vi "Load Selected File Format Class.vi"(8 "error in (no error)":errorcluster, 10 "Protocol in":string, 11 "Class Lookup":variant) -> (0 "error out":errorcluster, 2 "FileFormat.lvclass":refnum<class "FileFormat.lvclass">, 3 "Class Lookup":variant)   [LabVIEW 2013, in "Engine Simulation Toolkit System Explorer.lvlib"]
uses:
  Engine Simulation Toolkit System Explorer.lvlib
  File Formats.lvlibp/Parent/FileFormat.lvclass
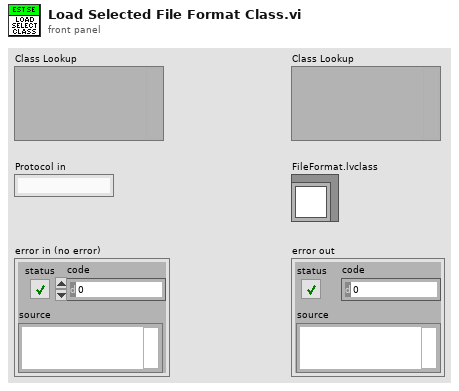
[diagram p1: front panel]
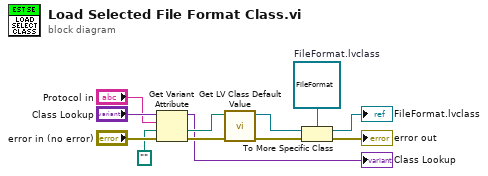
[diagram p0: block diagram]
diagram:
  w11 = refnum<class "FileFormat.lvclass"> refnum  # FileFormat.lvclass
  n1 = Get Variant Attribute(Variant="Class Lookup", name="Protocol in", default value (empty Variant)=path "", error in="error in (no error)") -> (duplicate Variant=→"Class Lookup":variant, value=w6:path, error out=w5:errorcluster)  [unwired: 1 out]
  n2 = call <vilib>:"Get LV Class Default Value.vi"("error in (no error)"=w5, "class path"=w6) -> ("error out"=w4:errorcluster, "object"=w3:refnum<class>)  [unwired: 8 in]
  n3 = To More Specific Class(target class=w11, reference=w3, error in=w4) -> (specific class reference=→"FileFormat.lvclass":refnum<class "FileFormat.lvclass">, error out=→"error out":errorcluster)
